vi "Trigger Logic FPGA.vi"(5 "Interlock on":bool, 7 "External trigger":bool) -> (3 "Triggered":bool)   [LabVIEW 2014]
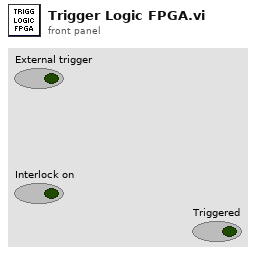
[diagram p1: front panel]
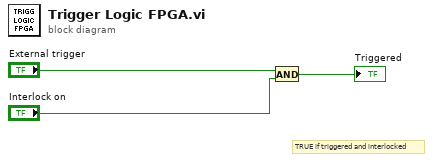
[diagram p0: block diagram]
diagram:
  # "TRUE if triggered and interlocked"
  n1 = And(x="External trigger", y="Interlock on") -> (x .and. y?=→"Triggered":bool)
